vi "Get Top Target Information.vi"(0 "Vision Info Array":dbl[][](array[numeric])) -> (1 "Center of Mass X":dbl, 2 "Bounding Box Width":dbl, 3 "Bounding Box Height":dbl, 4 "Calculated Shooter Speed":dbl)   [LabVIEW 2012]
uses:
  Globals/Shooter Testing.vi
panel:
  in  "Manual shooter testing?":bool
  in  "Manual shooter test speed":dbl
  # "Analysis"
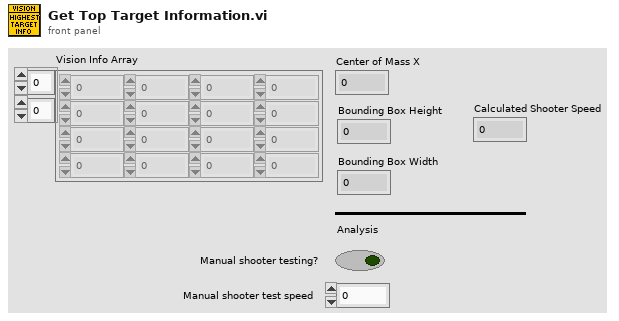
[diagram p1: front panel]
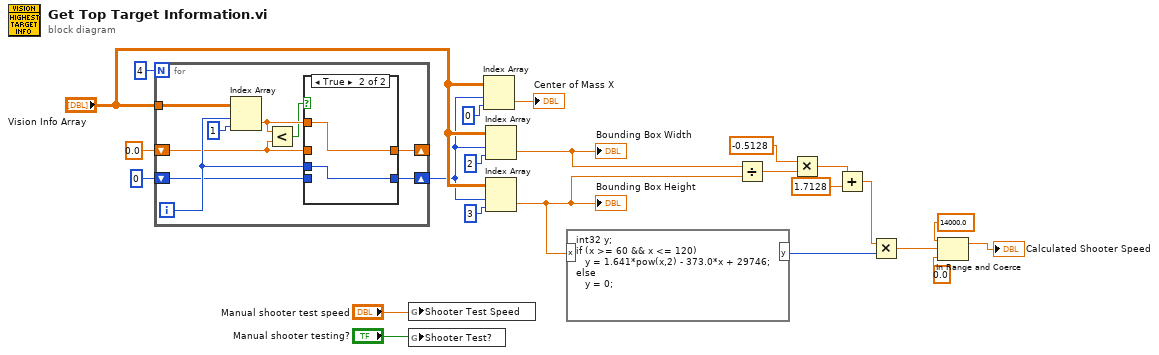
[diagram p0: block diagram]
diagram:
  n1 = for {
    N: 4 -> [_]
    tunnel: "Vision Info Array" -> [w32]
    shift-right: [w27] -> _
    shift-left: 0.0 ("Numeric") -> [w25]
    shift-right: [w29] -> w15
    shift-left: 0 -> [w26]
    i -> [w30]
    n2 = Index Array(array=w32, index (row)=w30, index (col)=1 ("disabled index (col)")) -> (element=w28:dbl)
    n3 = Less?(x=w28, y=w25) -> (x < y?=w24:bool)
    n4 = case shown="True" w24 {
      tunnel: w30 -> [_ w36]
      tunnel: [w34 w36] -> w29
      tunnel: w28 -> [_ w35]
      tunnel: [w33 w35] -> w27
      tunnel: w26 -> [w34 _]
      tunnel: w25 -> [w33 _]
      frame False {
      }
      frame True {
      }
    }
  }
  n5 = global write "Shooter Testing.vi" "Shooter Test Speed"("Manual shooter test speed") -> ()
  n6 = global write "Shooter Testing.vi" "Shooter Test?"("Manual shooter testing?") -> ()
  n7 = Index Array(array="Vision Info Array", index (row)=w15, index (col)=0) -> (element=→"Center of Mass X":dbl)
  n8 = Index Array(array="Vision Info Array", index (row)=w15, index (col)=2) -> (element=w12:dbl)
  "Bounding Box Width" <- w12
  n9 = Index Array(array="Vision Info Array", index (row)=w15, index (col)=3) -> (element=w11:dbl)
  "Bounding Box Height" <- w11
  n10 = formula code="int32 y;\nif (x >= 60 && x <= 120)\n   y = 1.641*pow(x,2) - 373.0*x + 29746;\nelse\n   y = 0;"("x"=w11) -> ("y"=w6:i32)
  n11 = Divide(x=w12, y=w11) -> (x/y=w10:dbl)
  n12 = Multiply(x=-0.5128, y=w10) -> (x*y=w8:dbl)
  n13 = Add(x=w8, y=1.7128) -> (x+y=w5:dbl)
  n14 = Multiply(x=w5, y=w6) -> (x*y=w4:dbl)
  n15 = In Range and Coerce(upper limit=14000.0, x=w4, lower limit=0.0) -> (coerced(x)=→"Calculated Shooter Speed":dbl)  [unwired: 1 out]
